vi "RP Write Command VISA.vi"(7 "Config offset":u64, 8 "Error In":errorcluster, 9 "Command payload":u64 format="%x", 10 "Command number":T1, 11 "VISA resource":refnum<visa-resource-name>) -> (0 "Error Out":errorcluster, 2 "bytes written":i32, 3 "VISA resource out":refnum<visa-resource-name>)   [LabVIEW 2015]
uses:
  RP Command.ctl
panel:
  out "x .or. y?":u64 format="%x"
  out "x << y":u64 format="%x"
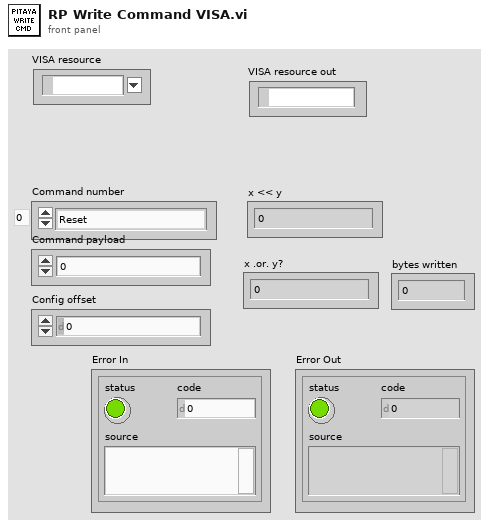
[diagram p1: front panel]
types:
  T1 = typedef "RP Command.ctl" = enum16{"Reset", "Read IDN", "Stop server", "Get status", "Get temperature", "Connect client", "Arm", "Software trigger", "Get whole buffer", "Get chunk", "System call", "Get config", "Set config", "Recieve data", "Play pattern", "Transmit data"}
  T2 = enum16{"big-endian, network order", "native, host order", "little-endian"}
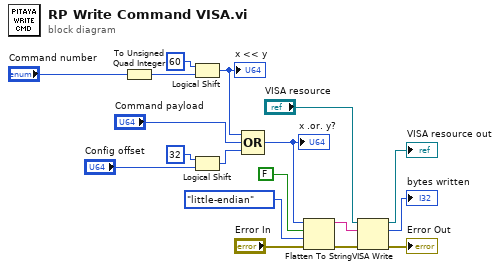
[diagram p0: block diagram]
diagram:
  n1 = To Unsigned Quad Integer(1:"Command number") -> (0:w10:u64)
  n2 = Logical Shift(y=i16 60, x=w10) -> (x << y=w16:u64)
  "x << y" <- w16
  n3 = Logical Shift(y=i16 32, x="Config offset") -> (x << y=w7:u64)
  n4 = Compound Arithmetic op=OR(w16, "Command payload", w7) -> (w11:u64)
  "x .or. y?" <- w11
  n5 = Flatten To String(anything=w11, prepend array or string size? (T)=FALSE, byte order (0:big-endian, network order)=T2."little-endian", error in (no error)="Error In") -> (data string=w2:string, error out=w4:errorcluster)  [unwired: 1 out]
  n6 = VISA Write(VISA resource name="VISA resource", write buffer=w2, error in (no error)=w4) -> (VISA resource name out=→"VISA resource out":refnum<visa-resource-name>, return count=→"bytes written":u32, error out=→"Error Out":errorcluster)
